vi "Counter.vi"(8 "error in":errorcluster caption="错误输入", 11 "Enum":enum16{"Init", "Start", "Read", "Stop", "Clear"}(ring)) -> (0 "error out":errorcluster caption="错误输出", 3 "data":dbl format="%0.2f")   [LabVIEW 2024]
uses:
  <vilib>/DAQmx/read.llb/DAQmx Read (Counter DBL 1Chan 1Samp).vi
  <vilib>/DAQmx/create/channels.llb/DAQmx Create Channel (CI-Position-Angular Encoder).vi
  <vilib>/DAQmx/miscellaneous.llb/DAQmx Fill In Error Info.vi
  <resource>/objmgr/daqmx.rc
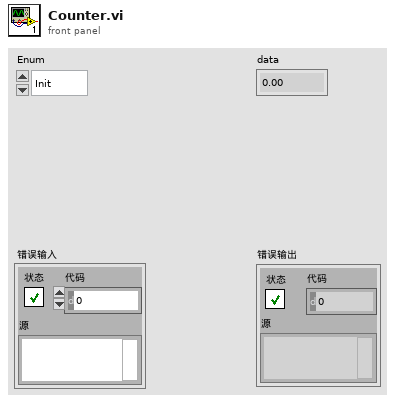
[diagram p1: front panel]
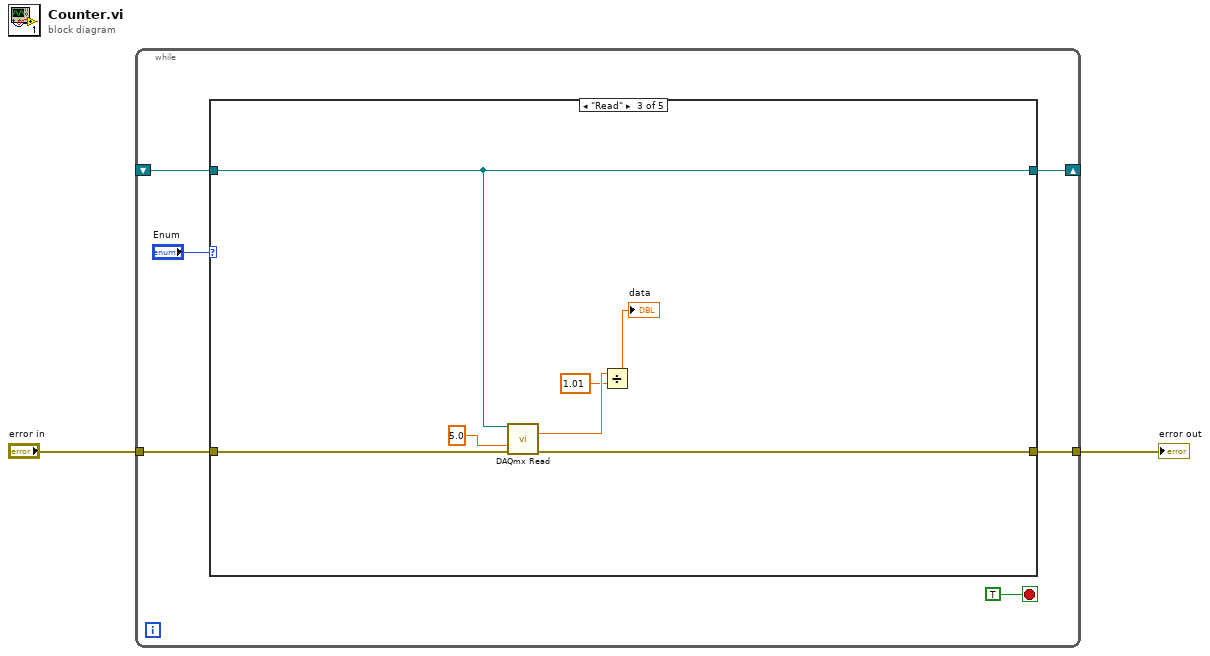
[diagram p0: block diagram]
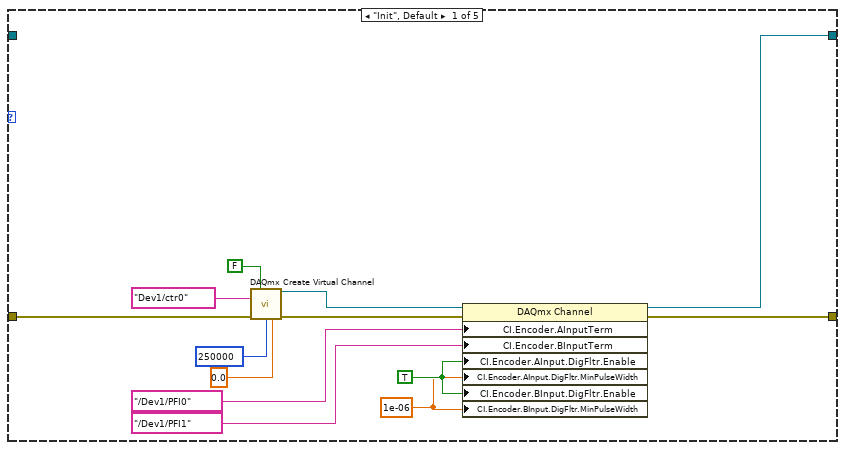
[diagram p2: hidden frame]
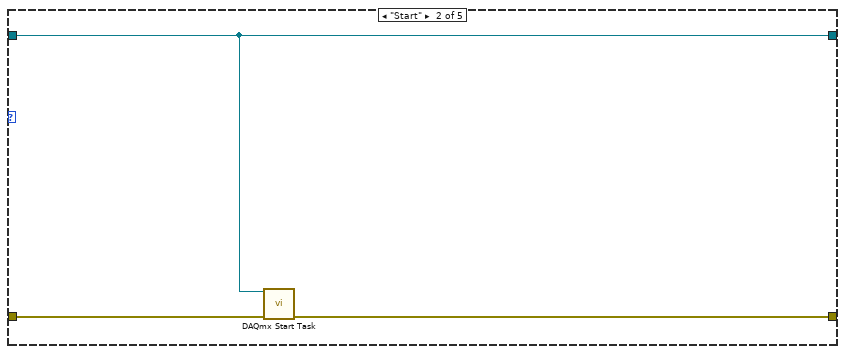
[diagram p3: hidden frame]
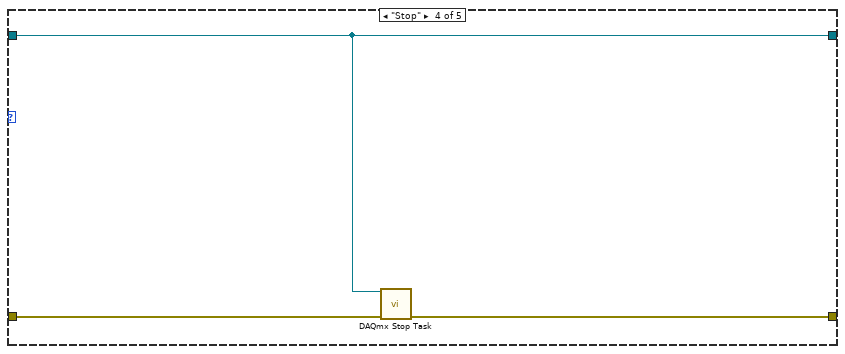
[diagram p4: hidden frame]
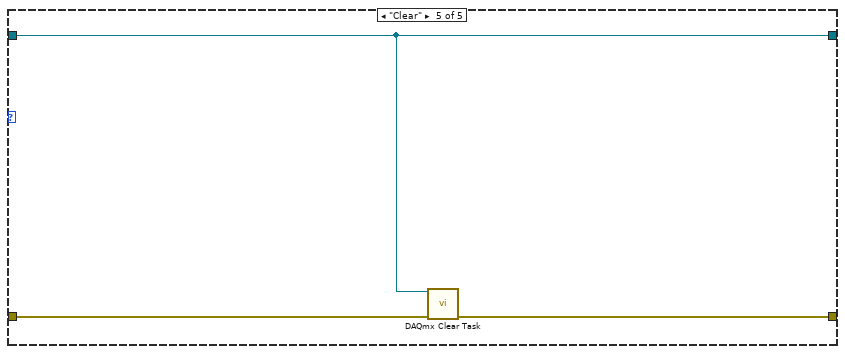
[diagram p5: hidden frame]
diagram:
  n1 = while {
    tunnel: "error in" -> [w8]
    tunnel: [w6] -> w1
    shift-right: [w7] -> _
    shift-left: _ -> [w4]
    stop <- TRUE stop-if-true
    n2 = case shown="\"Read\"" "Enum" {
      tunnel: w8 -> [w21 w24 w30 w33 w37]
      tunnel: [w14 w22 w28 w34 w35] -> w7
      tunnel: [w13 w23 w29 w32 w36] -> w6
      tunnel: w4 -> [_ w22 w28 w34 w35]
      frame "Init", Default {
        w10 = 1e-06 ("CI.Encoder.AInput.DigFltr.MinPulseWidth")
        w11 = TRUE ("CI.Encoder.AInput.DigFltr.Enable")
        n3 = call-poly <vilib>:"DAQmx Create Virtual Channel.vi"("z index enable"=FALSE ("启用Z索引"), "counter"=tag "Dev1/ctr0" ("计数器"), "error in"=w21, "pulses per revolution"=u32 250000 ("脉冲每转"), "initial angle"=0.0) -> ("task out"=w19:refnum<k21>, "error out"=w17:errorcluster)  [unwired: 9 in]
        n4 = property class="DAQmx Channel"(reference=w19, error in=w17, "CI.Encoder.AInputTerm"=tag "/Dev1/PFI0" ("输入接线端"), "CI.Encoder.BInputTerm"=tag "/Dev1/PFI1" ("B输入接线端"), "CI.Encoder.AInput.DigFltr.Enable"=w11, "CI.Encoder.AInput.DigFltr.MinPulseWidth"=w10, "CI.Encoder.BInput.DigFltr.Enable"=w11, "CI.Encoder.BInput.DigFltr.MinPulseWidth"=w10) -> (reference out=w14:refnum<k21>, error out=w13:errorcluster)
      }
      frame "Start" {
        n5 = call <vilib>:"DAQmx Start Task.vi"("task/channels in"=w22, "error in"=w24) -> ("error out"=w23:errorcluster)  [unwired: 12 in, 1 out]
      }
      frame "Read" {
        n6 = call-poly <vilib>:"DAQmx Read.vi"("task/channels in"=w28, "timeout"=5.0, "error in"=w30) -> ("data"=w26:dbl, "error out"=w29:errorcluster)  [unwired: 10 in, 1 out]
        n7 = Divide(x=w26, y=1.01) -> (x/y=→"data":dbl)
      }
      frame "Stop" {
        n8 = call <vilib>:"DAQmx Stop Task.vi"("task/channels in"=w34, "error in"=w33) -> ("error out"=w32:errorcluster)  [unwired: 12 in, 1 out]
      }
      frame "Clear" {
        n9 = call <vilib>:"DAQmx Clear Task.vi"("task in"=w35, "error in"=w37) -> ("error out"=w36:errorcluster)  [unwired: 13 in]
      }
    }
  }
  "error out" <- w1
